vi "Initialize.vi"(8 "error in (no error)":errorcluster, 9 "ID Query (T: Check)":bool=TRUE, 10 "Reset (T: Reset)":bool=TRUE, 11 "Yokogawa WT2X0 in":refnum<class "Yokogawa WT2X0.lvclass">) -> (0 "error out":errorcluster, 2 "VISA resource name":refnum<visa-resource-name>, 3 "Yokogawa WT2X0 out":refnum<class "Yokogawa WT2X0.lvclass">)   [LabVIEW 2014, in "Generic Power Analyzer.lvlib" / "Yokogawa WT2X0.lvlib" / "Yokogawa WT2X0.lvclass"]
uses:
  Yokogawa WT2X0.lvclass
  Generic Power Analyzer/Generic Power Analyzer.lvclass
  <instrlib>/Yokogawa WT200 Series/Yokogawa WT200 Series.lvlib
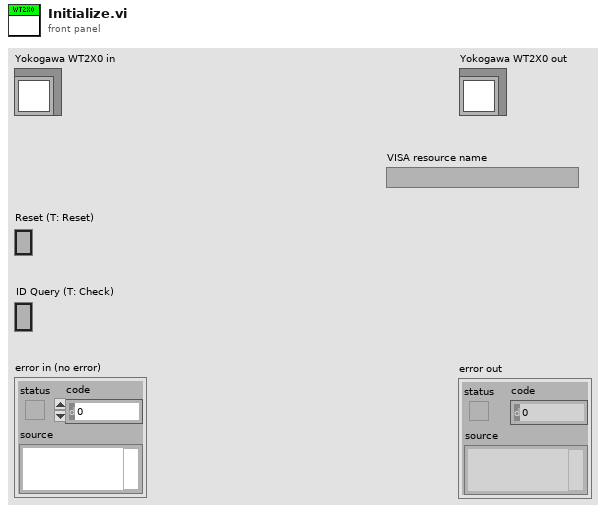
[diagram p1: front panel]
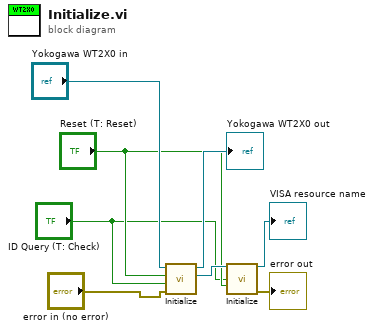
[diagram p0: block diagram]
diagram:
  n1 = call-parent <instrlib>:"Initialize.vi"("error in (no error)"="error in (no error)", "ID Query"="ID Query (T: Check)", "Reset"="Reset (T: Reset)", "Generic Power Analyzer in"="Yokogawa WT2X0 in") -> ("VISA resource name"=w6:refnum<visa-resource-name>, "Generic Power Analyzer out"=→"Yokogawa WT2X0 out":refnum<class "Yokogawa WT2X0.lvclass">)  [unwired: 5 in, 1 out]
  n2 = call <instrlib>:"Initialize.vi"("VISA resource name"=w6, "ID Query (T: Check)"="ID Query (T: Check)", "Reset (T: Reset)"="Reset (T: Reset)") -> ("VISA resource name out"=→"VISA resource name":refnum<visa-resource-name>, "error out"=→"error out":errorcluster)  [unwired: 11 in]
